vi "CRYPEAQ Loudness.vi"(7 "ITU-R/SC?":bool, 8 "Nc":i32, 9 "fc":dbl[](array[numeric]), 10 "Ehs":dbl[](array[numeric]) format="%#.6f") -> (3 "Ntotal":dbl)   [LabVIEW 2013]
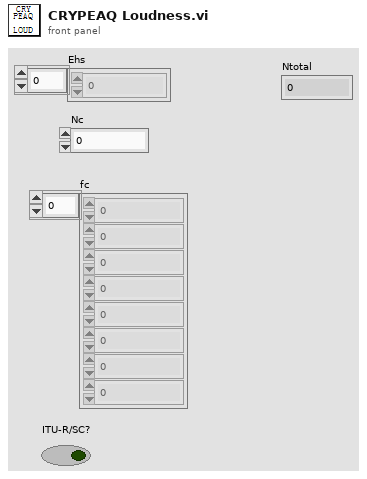
[diagram p1: front panel]
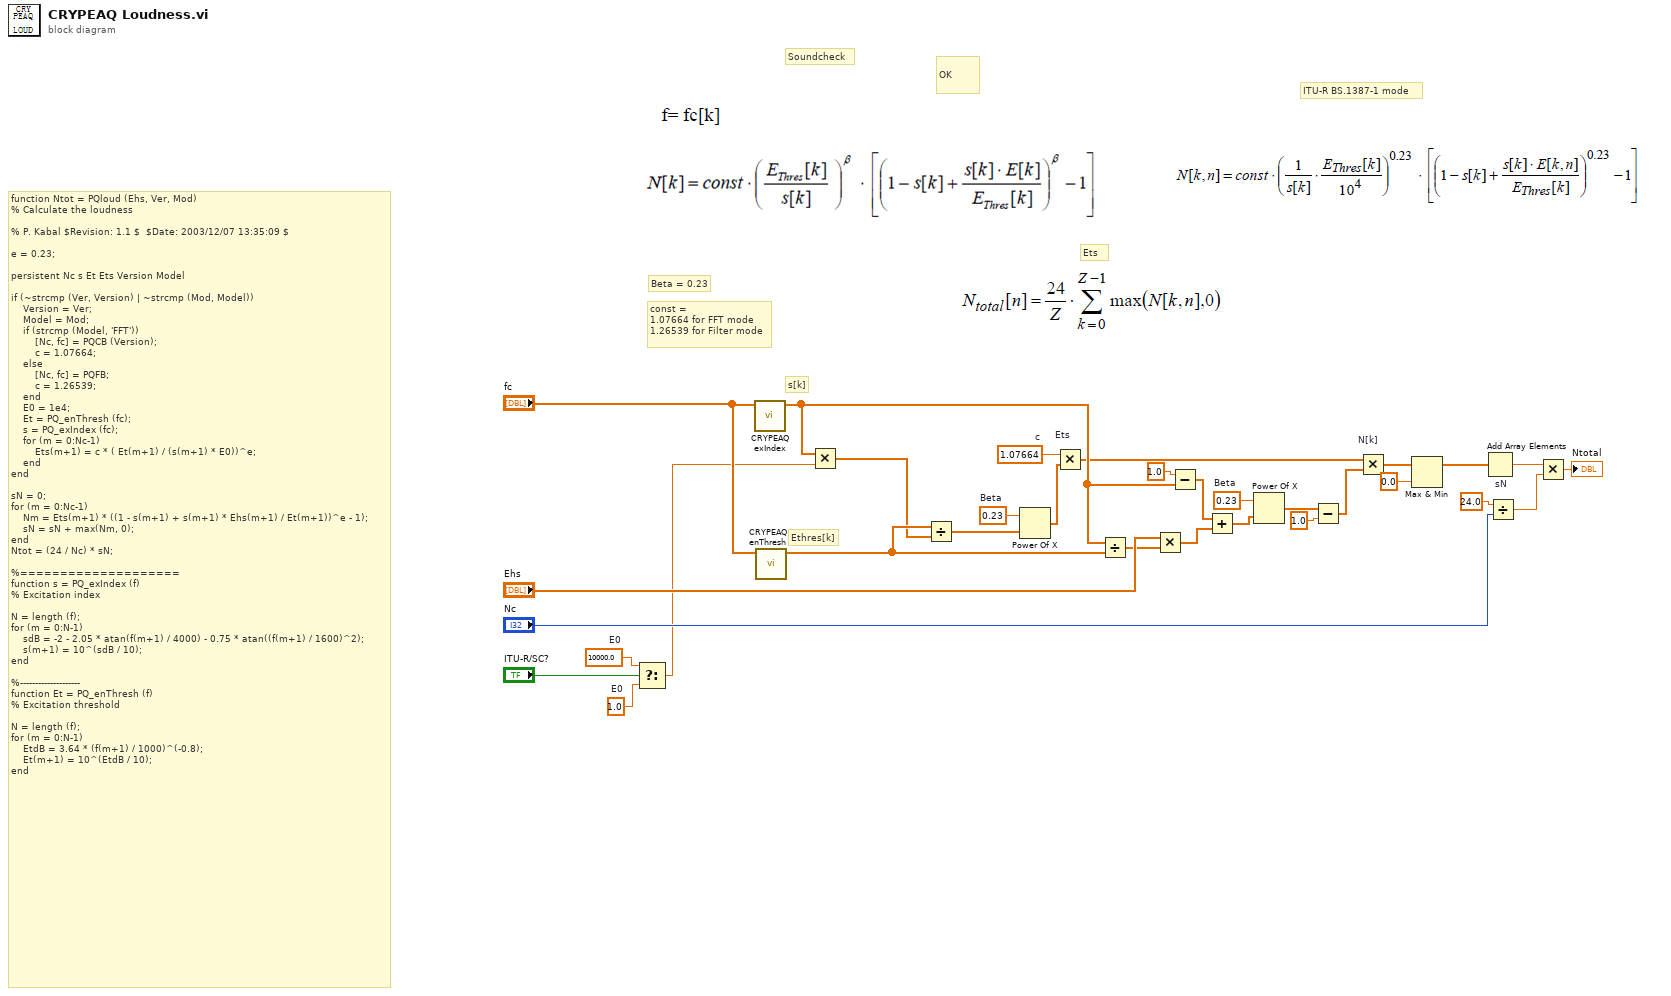
[diagram p0: block diagram]
diagram:
  w3 = 10000.0  # E0
  w2 = 1.0  # E0
  w18 = 0.23  # Beta
  w8 = 1.07664  # c
  w29 = 0.23  # Beta
  # "OK"
  # "Ethres[k]"
  # "s[k]"
  # "const = \n1.07664 for FFT mode\n1.26539 for Filter mode"
  # "Beta = 0.23"
  # "Ets"
  # "Soundcheck"
  # "ITU-R BS.1387-1 mode"
  # "function Ntot = PQloud (Ehs, Ver, Mod)\n% Calculate the loudness\n\n% P. Kabal $Revision: 1.1 $  $Date: 2003/12/07 13:35:09 $\n\ne = 0.23;\n\npersistent Nc s Et Ets Version Model\n\nif (~strcmp (Ver, Version) | ~strcmp (Mod, Model))\n    Version = Ver;\n    Model = Mod;\n    if (strcmp (Model, 'FFT'))\n        [Nc, fc] = PQCB (Version);\n        c = 1.07664;\n    else\n        [Nc, fc] = PQFB;\n        c = 1.26539;\n    end\n    E0 = 1e4;\n    Et = PQ_enThresh (fc);\n    s = PQ_exIndex (fc);\n    for (m = 0:Nc-1)\n        Ets(m+1) = c * ( Et(m+1) / (s(m+1) * E0))^e;\n    end\nend\n\nsN = 0;\nfor (m = 0:Nc-1)\n    Nm = Ets(m+1) * ((1 - s(m+1) + s(m+1) * Ehs(m+1) / Et(m+1))^e - 1);\n    sN = sN + max(Nm, 0);\nend\nNtot = (24 / Nc) * sN;\n\n%====================\nfunction s = PQ_exIndex (f)\n% Excitation index\n\nN = length (f);\nfor (m = 0:N-1)\n    sdB = -2 - 2.05 * atan(f(m+1) / 4000) - 0.75 * atan((f(m+1) / 1600)^2);\n    s(m+1) = 10^(sdB / 10);\nend\n\n%--------------------\nfunction Et = PQ_enThresh (f)\n% Excitation threshold\n\nN = length (f);\nfor (m = 0:N-1)\n    EtdB = 3.64 * (f(m+1) / 1000)^(-0.8);\n    Et(m+1) = 10^(EtdB / 10);\nend"
  n1 = Select(t=w3, s="ITU-R/SC?", f=w2) -> (s? t:f=w1:dbl)
  n2 = call "CRYPEAQ exIndex.vi"("f"="fc") -> ("s(Excitation index)"=w19:dbl[])  [unwired: 10 in]
  n3 = call "CRYPEAQ enThresh.vi"("f"="fc") -> ("Et(thres)"=w7:dbl[])  [unwired: 10 in]
  n4 = Multiply(x=w19, y=w1) -> (x*y=w5:dbl[])
  n5 = Divide(x=w7, y=w5) -> (x/y=w6:dbl[])
  n6 = Power Of X(1:w6, 2:w18) -> (0:w17:dbl[])
  n7 = Multiply "Ets"(x=w8, y=w17) -> (x*y=w16:dbl[])
  n8 = Divide(x=w19, y=w7) -> (x/y=w21:dbl[])
  n9 = Multiply(x="Ehs", y=w21) -> (x*y=w28:dbl[])
  n10 = Subtract(x=1.0 ("-x"), y=w19) -> (x-y=w23:dbl[])
  n11 = Add(x=w23, y=w28) -> (x+y=w25:dbl[])
  n12 = Power Of X(1:w25, 2:w29) -> (0:w24:dbl[])
  n13 = Subtract(x=w24, y=1.0 ("-x")) -> (x-y=w20:dbl[])
  n14 = Multiply "N[k]"(x=w16, y=w20) -> (x*y=w15:dbl[])
  n15 = Max & Min(x=w15, y=0.0 ("-x")) -> (max(x,y)=w13:dbl[])  [unwired: 1 out]
  n16 = Add Array Elements "sN"(numeric array=w13) -> (sum=w10:dbl)
  n17 = Divide(x=24.0, y="Nc") -> (x/y=w9:dbl)
  n18 = Multiply(x=w10, y=w9) -> (x*y=→"Ntotal":dbl)
